vi "close.vi"(0 "Enable":bool=TRUE, 5 "error in (no error)":errorcluster) -> (18 "YES":bool, 19 "error out":errorcluster)   [LabVIEW 2019]
doc: "Displays a standard dialog box that prompts users to enter information, such as a user name and password.\n--------------------\n\nThis Express VI is configured as follows:\n\nMessage to Display to the User:Do you realy want to close application?\nThe inputs are:"
panel:
  out "String":string="Do you realy want to close application?"
  in  "Cancel":bool
  in  "OK2":bool
  in  "OK1":bool
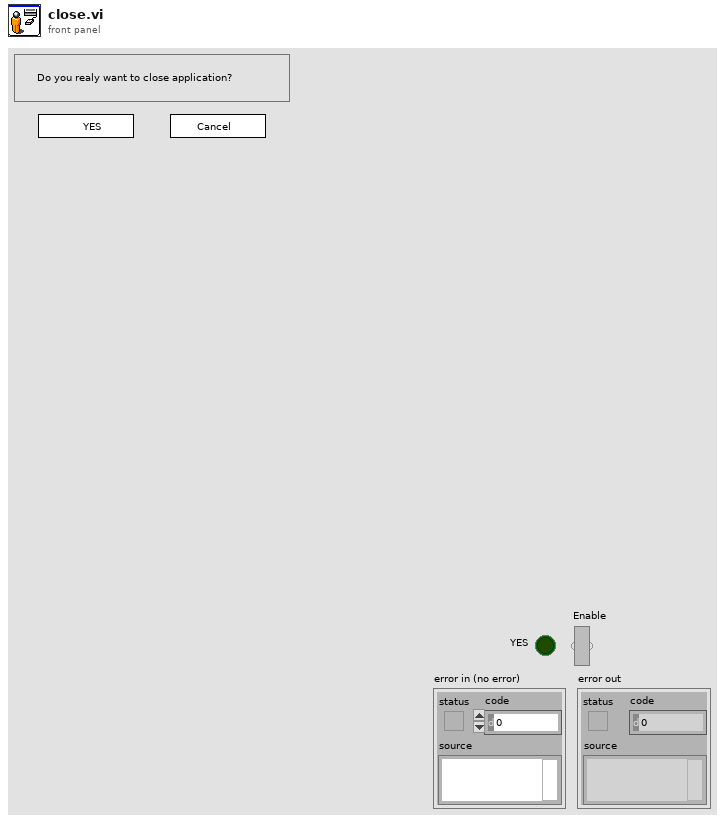
[diagram p1: front panel]
types:
  T1 = cluster{"Input Name":string, "Input Data Type":i32}[]
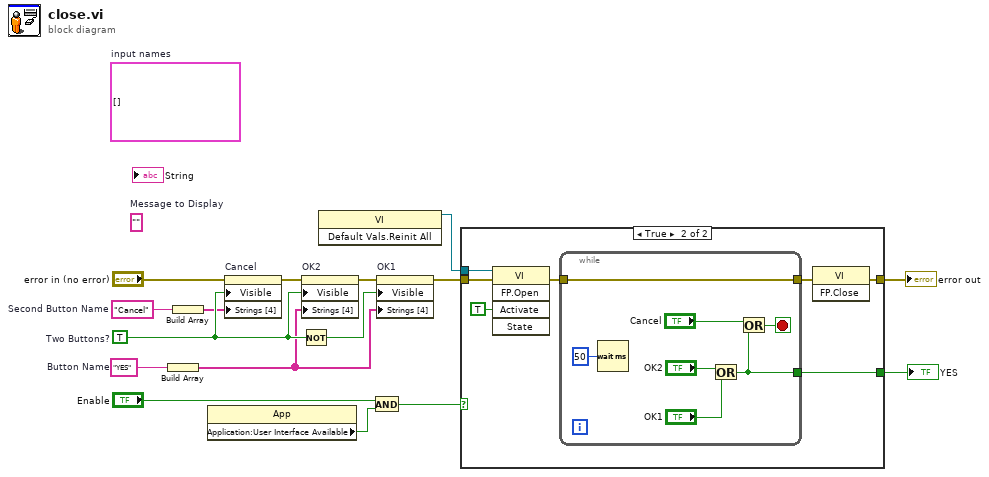
[diagram p0: block diagram]
diagram:
  (unwired) T1 []  # input names
  w10 = "Cancel"  # Second Button Name
  w8 = "YES"  # Button Name
  (unwired) ""  # Message to Display
  w16 = TRUE  # Two Buttons?
  n1 = Build Array(w8) -> (w9:string[])
  n2 = Build Array(w10) -> (w11:string[])
  n3 = property class="App"() -> ("Application:User Interface Available"=w3:bool)  [unwired: 2 in, 2 out]
  n4 = property on="Cancel" class="Bool"(error in="error in (no error)", "Visible"=w16, "Strings [4]"=w11) -> (error out=w13:errorcluster)  [unwired: 1 in, 1 out]
  n5 = Not(x=w16) -> (.not. x?=w14:bool)
  n6 = property on="OK2" class="Bool"(error in=w13, "Visible"=w16, "Strings [4]"=w9) -> (error out=w12:errorcluster)  [unwired: 1 in, 1 out]
  n7 = invoke class="VI" method="Default Vals.Reinit All"() -> (reference out=w2:refnum<vi>)  [unwired: 3 in, 2 out]
  n8 = And(x="Enable", y=w3) -> (x .and. y?=w1:bool)
  n9 = property on="OK1" class="Bool"(error in=w12, "Visible"=w14, "Strings [4]"=w9) -> (error out=w7:errorcluster)  [unwired: 1 in, 1 out]
  n10 = case shown="True" w1 {
    tunnel: [_ w24] -> w15
    tunnel: w7 -> [w17 w23]
    tunnel: [w17 w22] -> w5
    tunnel: w2 -> [_ w21]
    frame False {
    }
    frame True {
      n11 = invoke class="VI" method="FP.Open"(reference=w21, error in=w23, "Activate"=TRUE ("Activate?")) -> (error out=w19:errorcluster)  [unwired: 2 in, 4 out]
      n12 = while "Main While Loop" {
        tunnel: [w28] -> w24
        tunnel: w19 -> [w25]
        tunnel: [w25] -> w18
        stop <- w26 stop-if-true
        n13 = Wait (ms)(milliseconds to wait=u32 50 ("millisecond multiple")) -> ()  [unwired: 1 out]
        n14 = Or(x="OK2", y="OK1") -> (x .or. y?=w28:bool)
        n15 = Or(x="Cancel", y=w28) -> (x .or. y?=w26:bool)
      }
      n16 = invoke class="VI" method="FP.Close"(error in=w18) -> (error out=w22:errorcluster)  [unwired: 2 in, 2 out]
    }
  }
  "YES" <- w15
  "error out" <- w5
